vi "Gear Lift Intake.vi"(8 "Release":bool, 10 "Exit Button":bool, 11 "Trigger":bool) -> ()   [LabVIEW 2016]
uses:
  <vilib>/Rock Robotics/Network Tables/NT Write Boolean.vi
  Robot Global Data.vi
  <vilib>/Rock Robotics/WPI/Solenoid/WPI_SolenoidSetEnum.vi
  <vilib>/Rock Robotics/WPI/Solenoid/Deprecated/WPI_SolenoidGetBool.vi
panel:
  in  "Gear Grab Delay":dbl=0.01
  in  "State Count 2":dbl=1.0
  in  "Lift Latch":bool
  in  "Grab Open Delay":dbl=0.58
  out "Case Status":dbl
  in  "Grab Stat":bool
  in  "Lift Stat":bool
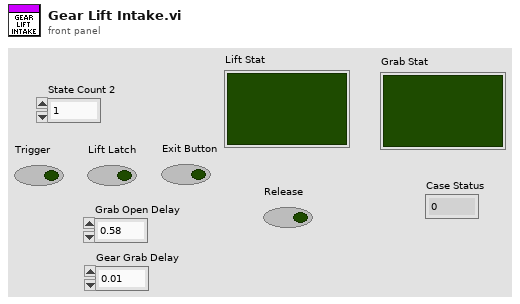
[diagram p1: front panel]
types:
  T1 = typedef "WPI_SwitchDevRef.ctl" = cluster{"DevStatus":errorcluster, "DIO Channel":T2, "CntIndex":T3, "Normally Closed":bool}
  T2 = typedef "FPGA_DIOChannel.ctl" = enum8{"DIO 0", "DIO 1", "DIO 2", "DIO 3", "DIO 4", "DIO 5", "DIO 6", "DIO 7", "DIO 8", "DIO 9", "DIO MXP 0", "DIO MXP 1", "DIO MXP 2", "DIO MXP 3", "DIO MXP 4", "DIO MXP 5", "DIO MXP 6", "DIO MXP 7", "DIO MXP 8", "DIO MXP 9", "DIO MXP 10", "DIO MXP 11", "DIO MXP 12", "DIO MXP 13", "DIO MXP 14", "DIO MXP 15", "SPI Port CS1", "SPI Port CS2", "SPI Port CS3", "SPI Port MISO", "SPI Port MOSI", "Invalid"}
  T3 = typedef "FPGA_CounterCtrSystemIndex.ctl" = enum8{"Ctr 0", "Ctr 1", "Ctr 2", "Ctr 3", "Ctr 4", "Ctr 5", "Ctr 6", "Ctr 7", "Invalid"}
  T4 = typedef "WPI_SolenoidDevRef.ctl" = cluster{"DevStatus":errorcluster, "Pneumatics Control Module":u8, "Forward Solenoid Channel":T5, "Reverse Solenoid Channel":T5}
  T5 = typedef "WPI_SolenoidChannel.ctl" = enum8{"Solenoid 0", "Solenoid 1", "Solenoid 2", "Solenoid 3", "Solenoid 4", "Solenoid 5", "Solenoid 6", "Solenoid 7", "Invalid"}
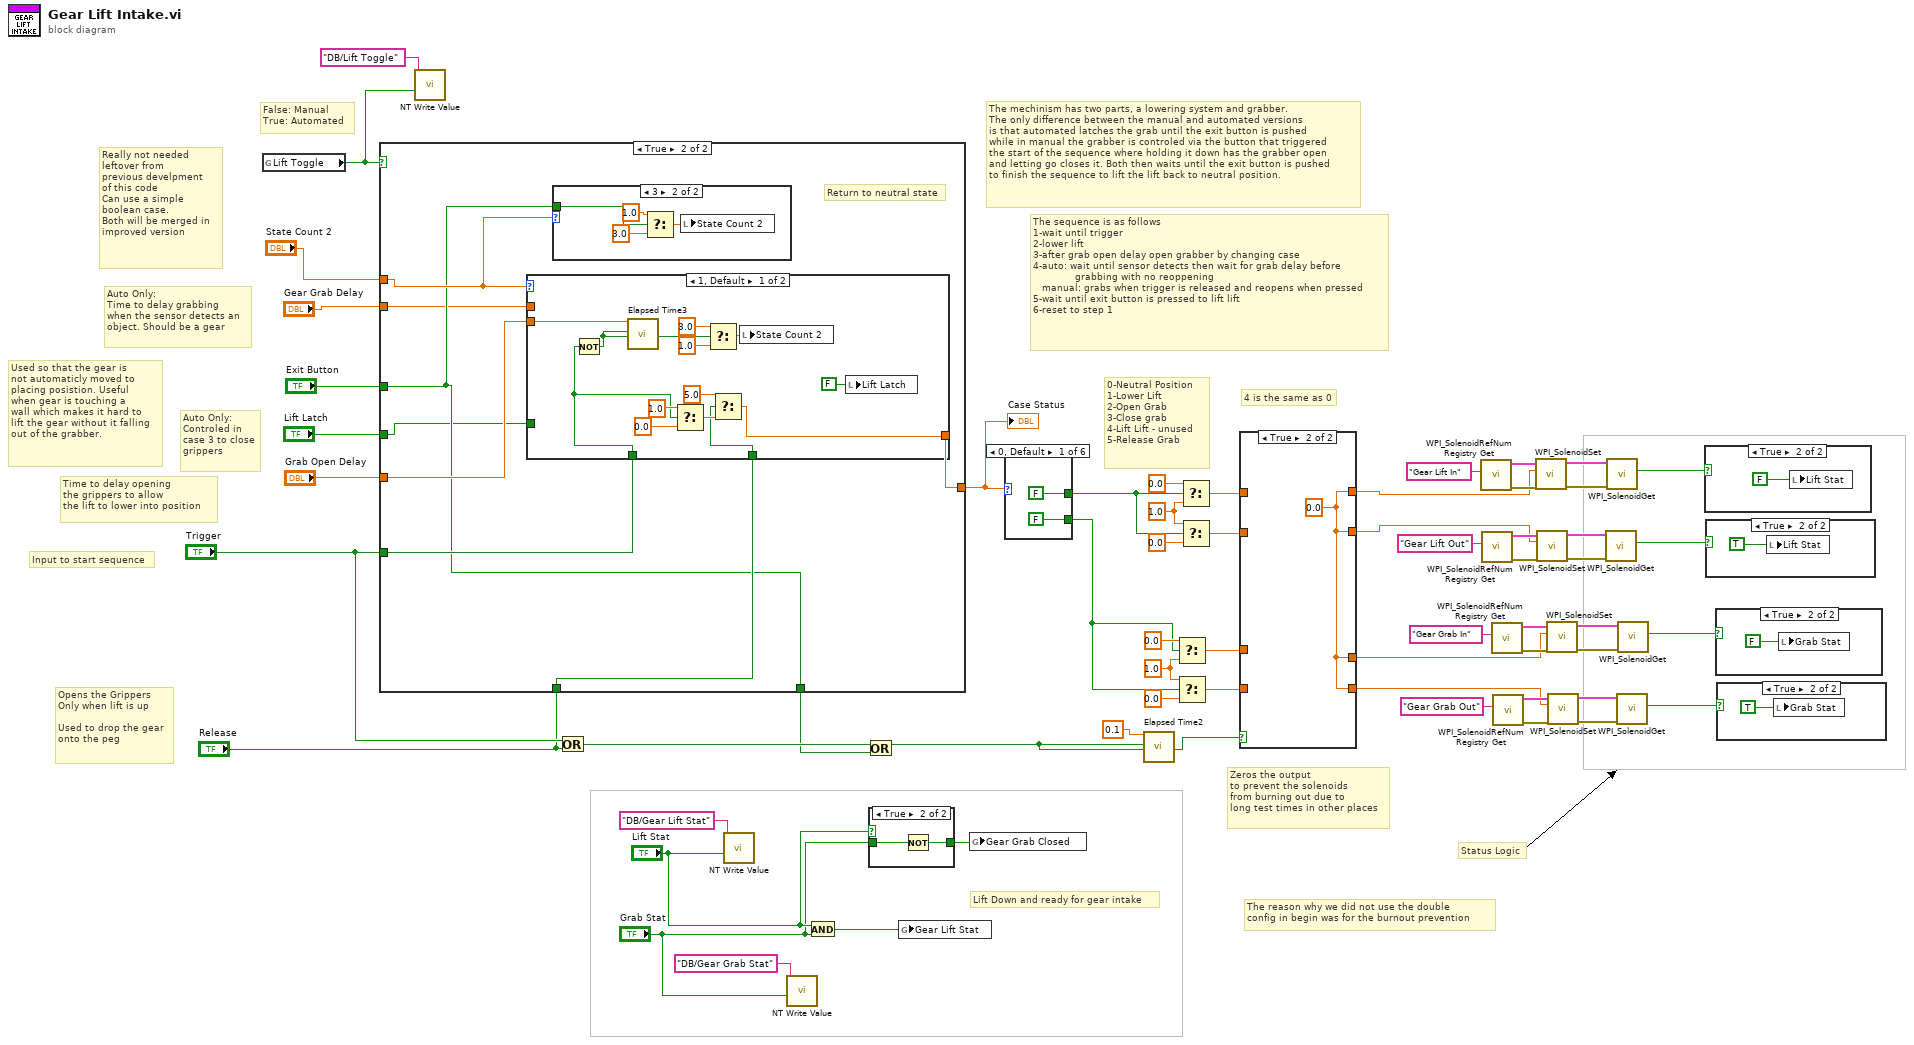
[diagram p0: block diagram]
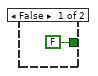
[diagram p2: hidden frame]
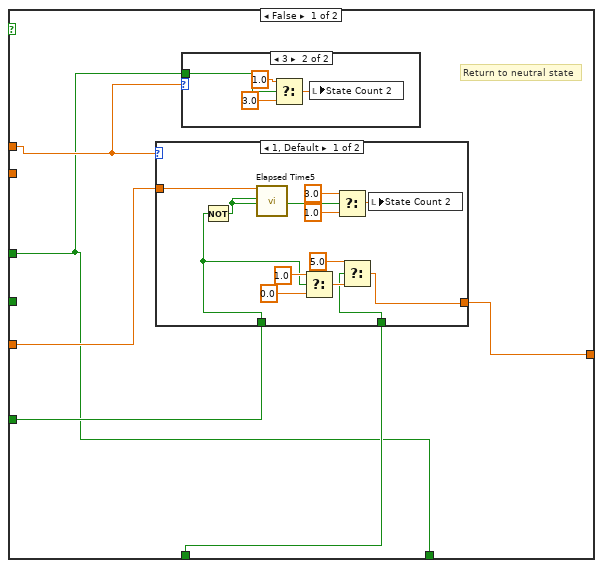
[diagram p3: hidden frame]
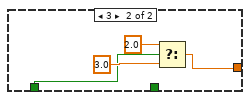
[diagram p5: hidden frame]
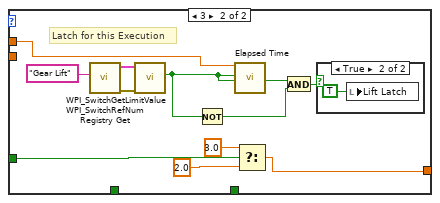
[diagram p7: hidden frame]
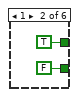
[diagram p14: hidden frame]
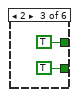
[diagram p15: hidden frame]
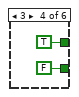
[diagram p16: hidden frame]
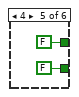
[diagram p17: hidden frame]
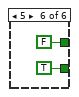
[diagram p18: hidden frame]
diagram:
  w26 = 1.0 ("f")
  w51 = 1.0 ("f")
  # "The sequence is as follows\n1-wait until trigger\n2-lower lift\n3-after grab open delay open grabber by changing case\n4-auto: wait until sensor detects then wait for grab delay before \n              grabbing with no reoppening\n   manual: grabs when trigger is released and reopens when pressed\n5-wait until exit button is pressed to lift lift\n6-reset to step 1"
  # "The reason why we did not use the double\nconfig in begin was for the burnout prevention"
  # "4 is the same as 0"
  # "The mechinism has two parts, a lowering system and grabber.\nThe only difference between the manual and automated versions\nis that automated latches the grab until the exit button is pushed \nwhile in manual the grabber is controled via the button that triggered\nthe start of the sequence where holding it down has the grabber open\nand letting go closes it. Both then waits until the exit button is pushed \nto finish the sequence to lift the lift back to neutral position."
  # "Zeros the output\nto prevent the solenoids\nfrom burning out due to\nlong test times in other places"
  # "Opens the Grippers\nOnly when lift is up\n\nUsed to drop the gear\nonto the peg"
  # "Input to start sequence"
  # "Time to delay opening\nthe grippers to allow\nthe lift to lower into position"
  # "Used so that the gear is \nnot automaticly moved to\nplacing posistion. Useful\nwhen gear is touching a \nwall which makes it hard to\nlift the gear without it falling\nout of the grabber."
  # "Auto Only:\nTime to delay grabbing \nwhen the sensor detects an\nobject. Should be a gear"
  # "Really not needed\nleftover from\nprevious develpment\nof this code\nCan use a simple\nboolean case.\nBoth will be merged in\nimproved version"
  # "Auto Only:\nControled in \ncase 3 to close\ngrippers"
  # "False: Manual\nTrue: Automated"
  # "Status Logic"
  # "Lift Down and ready for gear intake"
  # "0-Neutral Position\n1-Lower Lift\n2-Open Grab\n3-Close grab\n4-Lift Lift - unused \n5-Release Grab"
  n1 = global read "Robot Global Data.vi" "Lift Toggle"() -> (w11:bool)
  n2 = case shown="True" w11 {
    tunnel: "Trigger" -> [w66 w95]
    tunnel: [w67 w96] -> w15
    tunnel: "Release" -> [w65 w94]
    tunnel: "Grab Open Delay" -> [w63 w92]
    tunnel: "Lift Latch" -> [_ w90]
    tunnel: "Exit Button" -> [w62 w91]
    tunnel: [w62 w91] -> w6
    tunnel: "State Count 2" -> [w64 w93]
    tunnel: "Gear Grab Delay" -> [_ w89]
    frame False {
      # "Return to neutral state"
      n3 = case shown="1, Default" w64 {
        tunnel: [w75 w88] -> w67
        tunnel: w66 -> [w77 w85]
        tunnel: w65 -> [w73 _]
        tunnel: w63 -> [w72 _]
        frame 1, Default {
          n4 = Not(x=w77) -> (.not. x?=w84:bool)
          n5 = call "Elapsed Time5"("Time Target (s)"=w72, "Reset"=w84, "Auto Reset"=w84) -> ("Time has Elapsed"=w81:bool)  [unwired: 9 in, 7 out]
          n6 = Select(t=1.0, s=w77, f=0.0) -> (s? t:f=w76:dbl)
          n7 = Select(t=3.0, s=w81, f=1.0) -> (s? t:f=w80:dbl)
          n8 = Select(t=5.0, s=w73, f=w76) -> (s? t:f=w75:dbl)
          n9 = local write "State Count 2"(w80) -> ()
        }
        frame 3 {
          n10 = Select(t=2.0, s=w85, f=3.0) -> (s? t:f=w88:dbl)
        }
      }
      n11 = case shown="3" w64 {
        tunnel: w62 -> [_ w71]
        frame 1, Default {
        }
        frame 3 {
          n12 = Select(t=1.0, s=w71, f=3.0) -> (s? t:f=w68:dbl)
          n13 = local write "State Count 2"(w68) -> ()
        }
      }
    }
    frame True {
      # "Return to neutral state"
      n14 = case shown="1, Default" w93 {
        tunnel: [w105 w126] -> w96
        tunnel: w95 -> [w107 _]
        tunnel: w94 -> [w103 _]
        tunnel: w92 -> [w102 _]
        tunnel: w90 -> [_ w123]
        tunnel: w89 -> [_ w115]
        frame 1, Default {
          n15 = Not(x=w107) -> (.not. x?=w114:bool)
          n16 = call "Elapsed Time3"("Time Target (s)"=w102, "Reset"=w114, "Auto Reset"=w114) -> ("Time has Elapsed"=w111:bool)  [unwired: 9 in, 7 out]
          n17 = Select(t=1.0, s=w107, f=0.0) -> (s? t:f=w106:dbl)
          n18 = Select(t=3.0, s=w111, f=1.0) -> (s? t:f=w110:dbl)
          n19 = Select(t=5.0, s=w103, f=w106) -> (s? t:f=w105:dbl)
          n20 = local write "State Count 2"(w110) -> ()
          n21 = local write "Lift Latch"(FALSE ("Lift Latch")) -> ()
        }
        frame 3 {
          # "Latch for this Execution"
          n22 = call <vilib>:"WPI_SwitchRefNum Registry Get.vi"("refnum name"="Gear Lift") -> ("error out"=w118:errorcluster, "SwitchDevRef"=w117:T1)  [unwired: 9 in]
          n23 = call <vilib>:"WPI_SwitchGetLimitValue.vi"("error in (no error)"=w118, "SwitchDevRef"=w117) -> ("Switch Pressed"=w122:bool)  [unwired: 7 in, 2 out]
          n24 = Not(x=w122) -> (.not. x?=w121:bool)
          n25 = call "Elapsed Time"("Time Target (s)"=w115, "Reset"=w122, "Auto Reset"=w122) -> ("Time has Elapsed"=w120:bool)  [unwired: 9 in, 7 out]
          n26 = Select(t=3.0, s=w123, f=2.0) -> (s? t:f=w126:dbl)
          n27 = And(x=w120, y=w121) -> (x .and. y?=w116:bool)
          n28 = case shown="True" w116 {
            frame False {
            }
            frame True {
              n29 = local write "Lift Latch"(TRUE ("Lift Latch")) -> ()
            }
          }
        }
      }
      n30 = case shown="3" w93 {
        tunnel: w91 -> [_ w100]
        frame 1, Default {
        }
        frame 3 {
          n31 = Select(t=1.0, s=w100, f=3.0) -> (s? t:f=w97:dbl)
          n32 = local write "State Count 2"(w97) -> ()
        }
      }
    }
  }
  "Case Status" <- w15
  n33 = call-poly <vilib>:"NT Write Value.vi"("Boolean"=w11, "Name"="DB/Lift Toggle") -> ()  [unwired: 9 in, 1 out]
  n34 = Or(x="Trigger", y="Release") -> (x .or. y?=w14:bool)
  n35 = call-poly <vilib>:"NT Write Value.vi"("Boolean"="Lift Stat", "Name"="DB/Gear Lift Stat") -> ()  [unwired: 9 in, 1 out]
  n36 = call-poly <vilib>:"NT Write Value.vi"("Boolean"="Grab Stat", "Name"="DB/Gear Grab Stat") -> ()  [unwired: 9 in, 1 out]
  n37 = And(x="Lift Stat", y="Grab Stat") -> (x .and. y?=w18:bool)
  n38 = Or(x=w14, y=w6) -> (x .or. y?=w7:bool)
  n39 = case shown="True" "Lift Stat" {
    tunnel: [FALSE w130] -> w3
    tunnel: "Grab Stat" -> [_ w129]
    frame False {
    }
    frame True {
      n40 = Not(x=w129) -> (.not. x?=w130:bool)
    }
  }
  n41 = global write "Robot Global Data.vi" "Gear Lift Stat"(w18) -> ()
  n42 = global write "Robot Global Data.vi" "Gear Grab Closed"(w3) -> ()
  n43 = case shown="0, Default" w15 {
    tunnel: [FALSE TRUE TRUE TRUE FALSE FALSE] -> w20
    tunnel: [FALSE FALSE TRUE FALSE FALSE TRUE] -> w19
    frame 0, Default {
    }
    frame 1 {
    }
    frame 2 {
    }
    frame 3 {
    }
    frame 4 {
    }
    frame 5 {
    }
  }
  n44 = call "Elapsed Time2"("Time Target (s)"=0.1, "Reset"=w7, "Auto Reset"=w7) -> ("Time has Elapsed"=w47:bool)  [unwired: 9 in, 7 out]
  n45 = Select(t=0.0, s=w19, f=w26) -> (s? t:f=w24:dbl)
  n46 = Select(t=w26, s=w19, f=0.0) -> (s? t:f=w22:dbl)
  n47 = Select(t=0.0, s=w20, f=w51) -> (s? t:f=w50:dbl)
  n48 = Select(t=w51, s=w20, f=0.0) -> (s? t:f=w49:dbl)
  n49 = case shown="True" w47 {
    tunnel: [w145 w147] -> w54
    tunnel: [w146 w147] -> w55
    tunnel: w50 -> [w146 _]
    tunnel: w49 -> [w145 _]
    tunnel: [w144 w147] -> w25
    tunnel: w24 -> [w144 _]
    tunnel: [w143 w147] -> w23
    tunnel: w22 -> [w143 _]
    frame False {
    }
    frame True {
      w147 = 0.0 ("f")
    }
  }
  n50 = call <vilib>:"WPI_SolenoidRefNum Registry Get.vi"("refnum name"="Gear Lift In") -> ("error out"=w61:errorcluster, "SolenoidDevRef"=w60:T4)  [unwired: 9 in]
  n51 = call <vilib>:"WPI_SolenoidRefNum Registry Get.vi"("refnum name"="Gear Lift Out") -> ("error out"=w58:errorcluster, "SolenoidDevRef"=w57:T4)  [unwired: 9 in]
  n52 = call <vilib>:"WPI_SolenoidRefNum Registry Get.vi"("refnum name"="Gear Grab In") -> ("error out"=w39:errorcluster, "SolenoidDevRef"=w38:T4)  [unwired: 9 in]
  n53 = call <vilib>:"WPI_SolenoidRefNum Registry Get.vi"("refnum name"="Gear Grab Out") -> ("error out"=w36:errorcluster, "SolenoidDevRef"=w35:T4)  [unwired: 9 in]
  n54 = call-poly <vilib>:"WPI_SolenoidSet.vi"("error in (no error)"=w61, "Value"=w55, "SolenoidDevRef"=w60) -> ("error out"=w46:errorcluster, "SolenoidDevRef"=w45:T4)  [unwired: 7 in]
  n55 = call-poly <vilib>:"WPI_SolenoidSet.vi"("error in (no error)"=w58, "Value"=w54, "SolenoidDevRef"=w57) -> ("error out"=w43:errorcluster, "SolenoidDevRef"=w44:T4)  [unwired: 7 in]
  n56 = call-poly <vilib>:"WPI_SolenoidSet.vi"("error in (no error)"=w39, "Value"=w25, "SolenoidDevRef"=w38) -> ("error out"=w33:errorcluster, "SolenoidDevRef"=w32:T4)  [unwired: 7 in]
  n57 = call-poly <vilib>:"WPI_SolenoidSet.vi"("error in (no error)"=w36, "Value"=w23, "SolenoidDevRef"=w35) -> ("error out"=w30:errorcluster, "SolenoidDevRef"=w31:T4)  [unwired: 7 in]
  n58 = call-poly <vilib>:"WPI_SolenoidGet.vi"("error in (no error)"=w43, "SolenoidDevRef"=w44) -> ("Value"=w40:bool)  [unwired: 7 in, 2 out]
  n59 = call-poly <vilib>:"WPI_SolenoidGet.vi"("error in (no error)"=w46, "SolenoidDevRef"=w45) -> ("Value"=w41:bool)  [unwired: 7 in, 2 out]
  n60 = call-poly <vilib>:"WPI_SolenoidGet.vi"("error in (no error)"=w30, "SolenoidDevRef"=w31) -> ("Value"=w28:bool)  [unwired: 7 in, 2 out]
  n61 = call-poly <vilib>:"WPI_SolenoidGet.vi"("error in (no error)"=w33, "SolenoidDevRef"=w32) -> ("Value"=w29:bool)  [unwired: 7 in, 2 out]
  n62 = case shown="True" w41 {
    frame False {
    }
    frame True {
      n63 = local write "Lift Stat"(FALSE ("Solinoid Stat")) -> ()
    }
  }
  n64 = case shown="True" w40 {
    frame False {
    }
    frame True {
      n65 = local write "Lift Stat"(TRUE ("Solinoid Stat")) -> ()
    }
  }
  n66 = case shown="True" w29 {
    frame False {
    }
    frame True {
      n67 = local write "Grab Stat"(FALSE ("Solinoid Stat")) -> ()
    }
  }
  n68 = case shown="True" w28 {
    frame False {
    }
    frame True {
      n69 = local write "Grab Stat"(TRUE ("Solinoid Stat")) -> ()
    }
  }
